vi "Excel Delete Unused Worksheets.vi"(0 "Sheets Ref In":refnum<k7>, 1 "Excel Ref In":refnum<k7>, 11 "Error In":errorcluster) -> (3 "Excel Ref Out":refnum<k7>, 4 "Sheets Ref Out":refnum<k7>, 15 "Error Out":errorcluster)   [LabVIEW 2013]
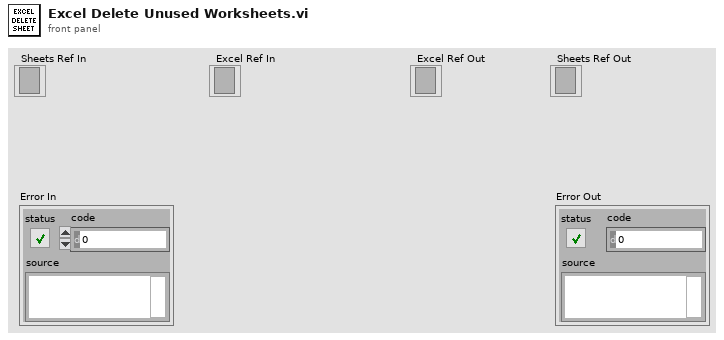
[diagram p1: front panel]
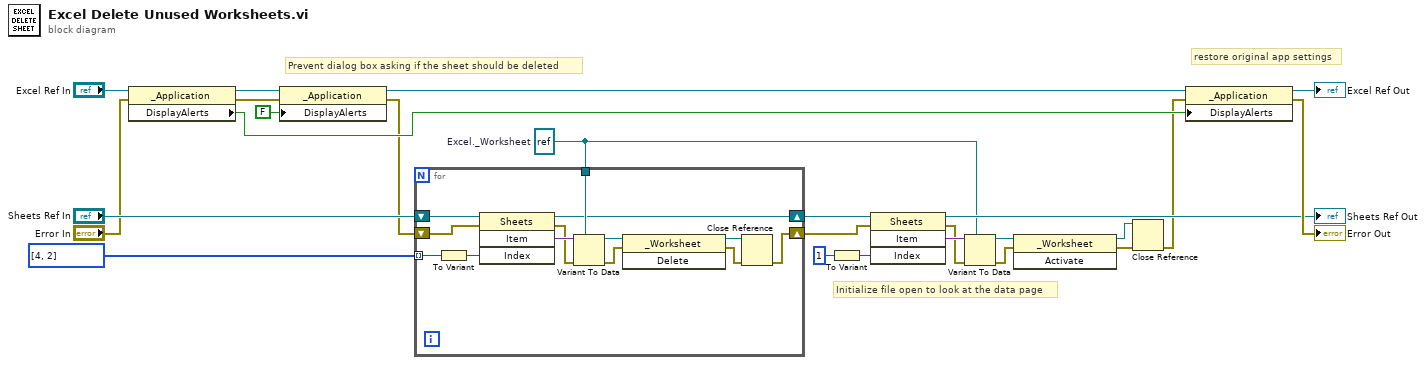
[diagram p0: block diagram]
diagram:
  w6 = refnum<k7> refnum  # Excel._Worksheet
  # "Initialize file open to look at the data page"
  # "restore original app settings"
  # "Prevent dialog box asking if the sheet should be deleted"
  n1 = property class="_Application"(reference="Excel Ref In", error in="Error In") -> (reference out=w21:refnum<k7>, error out=w22:errorcluster, "DisplayAlerts"=w15:bool)
  n2 = property class="_Application"(reference=w21, error in=w22, "DisplayAlerts"=FALSE) -> (reference out=w19:refnum<k7>, error out=w14:errorcluster)
  n3 = for {
    tunnel: w6 -> [w35]
    shift-right: [w30] -> w11
    shift-left: w14 -> [w38]
    shift-right: [w29] -> w10
    shift-left: "Sheets Ref In" -> [w34]
    tunnel: i32[] [4, 2] -> [w31] mode=indexing
    n4 = To Variant(anything=w31) -> (Variant=w36:variant)
    n5 = invoke class="Sheets" method="Item"(reference=w34, error in=w38, "Index"=w36) -> (reference out=w29:refnum<k7>, error out=w28:errorcluster, "Item"=w37:variant)  [unwired: 1 in, 1 out]
    n6 = Variant To Data(error in=w28, type=w35, Variant=w37) -> (data=w27:refnum<k7>, error out=w26:errorcluster)
    n7 = invoke class="_Worksheet" method="Delete"(reference=w27, error in=w26) -> (reference out=w33:refnum<k7>, error out=w32:errorcluster)  [unwired: 1 in, 1 out]
    n8 = Close Reference(reference=w33, error in (no error)=w32) -> (error out=w30:errorcluster)
  }
  n9 = To Variant(anything=1) -> (Variant=w13:variant)
  n10 = invoke class="Sheets" method="Item"(reference=w10, error in=w11, "Index"=w13) -> (reference out=→"Sheets Ref Out":refnum<k7>, error out=w5:errorcluster, "Item"=w8:variant)  [unwired: 1 in, 1 out]
  n11 = Variant To Data(error in=w5, type=w6, Variant=w8) -> (data=w7:refnum<k7>, error out=w4:errorcluster)
  n12 = invoke class="_Worksheet" method="Activate"(reference=w7, error in=w4) -> (reference out=w2:refnum<k7>, error out=w3:errorcluster)  [unwired: 1 in, 1 out]
  n13 = Close Reference(reference=w2, error in (no error)=w3) -> (error out=w1:errorcluster)
  n14 = property class="_Application"(reference=w19, error in=w1, "DisplayAlerts"=w15) -> (reference out=→"Excel Ref Out":refnum<k7>, error out=→"Error Out":errorcluster)
